vi "EQ_DATA_presort.vi"(8 "EQ Data and Report":u32[](array[numeric])=[2137719168, 671965161, 2137719168, 671965161, 2137719168, 671965161, 2137719168, 671965161, 2137719168, 671965161, 2137719168, 671965161, 2137719168, 671965161, 2137719168, 671965161, 2137719168, 671965161, 2137719168, 671965161, 2137719168, 671965161, 2137719168, 671965161, 2137719168, 671965161, 2137719168, 671965161, 2137719168, 671965161, 2137719168, 671965161, 2137719168, 671965161, 2137719168, 671965161, 2137719168, 671965161, 2137719168, 671965161, 2137719168, 671965161, 2137719168, 671965161, 2137719168, 671965161, 2137719168, 671965161, 2137719168, 671965161, 2137719168, 671965161, 2137719168, 671965161, 2137719168, 671965161, 2137719168, 671965161, 2137719168, 671965161, 2137719168, 671965161, 2137719168, 671965161, 2137719168, 671965161, 2137719168, 671965161, 2137719168, 671965161, 2137719168, 671965161, 2137719168, 671965161, 2137719168, 671965161, 2137719168, 671965161, 2137719168, 671965161, 2137719168, 671965161, 2137719168, 671965161, 2137719168, 671965161, 2137719168, 671965161, 2137719168, 671965161, 2137719168, 760049897, 2137719168, 491616745, 2137719168, 671965161, 2137719168, 671965161, 2137719168, 671965161, 2137719168, 671965161, 2137719168, 671965161, 2137719168, 671965161, 2137719168, 671965161, 2137719168, 671965161, 2137719168, 671965161, 2137719168, 671965161, 2137719168, 671965161, 2137719168, 671965161, 2137719168, 671965161, 2137719168, 671965161, 2137719168, 671965161, 2137719168, 671965161, 2137719168, 671965161, 2137719168, 671965161, 2137719168, 671965161, 2137719168, 671965161, 2137719168, 671965161, 2137719168, 671965161, 2137719168, 671965161, 2137719168, 671965161, 2137719168, 671965161, 2137719168, 671965161, 2137719168, 671965161, 2137719168, 671965161, 2137719168, 671965161, 2137719168, 671965161, 2137719168, 671965161, 2137719168, 671965161, 2137719168, 671965161, 2137719168, 671965161, 2137719168, 671965161, 2137719168, 671965161, 2137719168, 671965161, 2137719168, 671965161, 2137719168, 671965161, 2137719168, 671965161, 2137719168, 671965161, 2137719168, 671965161, 2137719168, 671965161, 2137719168, 671965161, 2137719168, 671965161, 2137719168, 671965161, 2137719168, 671965161, 2137719168, 671965161, 2137719168, 671965161, 2137719168, 671965161, 2137719168, 671965161, 2137719168, 671965161, 2137719168, 671965161, 2070610304, 671965161, 2070610304, 671965161, 2070610304, 671965161, 2070610304, 671965161, 2070610304, 671965161, 2070610304, 671965161, 2070610304, 671965161, 2070610304, 671965161, 2070610304, 671965161, 2070610304, 671965161, 2070610304, 671965161, 2070610304, 671965161, 2070610304, 671965161, 2070610304, 671965161, 2070610304, 671965161, 2070610304, 671965161, 2070610304, 671965161, 2070610304, 671965161, 2070610304, 671965161, 2070610304, 671965161, 2070610304, 671965161, 2070610304, 671965161, 2070610304, 671965161, 2070610304, 671965161, 2070610304, 671965161, 2070610304, 671965161, 2070610304, 671965161, 2070610304, 671965161, 2070610304, 671965161, 2070610304, 671965161, 2070610304, 671965161, 2070610304, 671965161, 2070610304, 671965161, 2070610304, 671965161, 2070610304, 671965161, 2070610304, 671965161, 2070610304, 671965161, 2070610304, 671965161, 2070610304, 671965161, 2070610304, 671965161, 2070610304, 671965161, 2070610304, 671965161, 2070610304, 671965161, 2070610304, 671965161, 2070610304, 671965161, 2070610304, 891148969, 2070610304, 1223555977, 2070610304, 671965161, 2070610304, 671965161, 2070610304, 671965161, 2070610304, 671965161, 2070610304, 671965161, 2070610304, 671965161, 2070610304, 671965161, 2070610304, 671965161, 2070610304, 671965161, 2070610304, 671965161, 2070610304, 671965161, 2070610304, 671965161, 2070610304, 671965161, 2070610304, 671965161, 2070610304, 671965161, 2070610304, 671965161, 2070610304, 671965161, 2070610304, 671965161, 2070610304, 671965161, 2070610304, 671965161, 2070610304, 671965161, 2070610304, 671965161, 2070610304, 671965161, 2070610304, 671965161, 2070610304, 671965161, 2070610304, 671965161, 2070610304, 671965161, 2070610304, 671965161, 2070610304, 671965161, 2070610304, 671965161, 2070610304, 671965161, 2070610304, 671965161, 2070610304, 671965161, 2070610304, 671965161, 2070610304, 671965161, 2070610304, 671965161, 2070610304, 671965161, 2070610304, 671965161, 2070610304, 671965161, 2070610304, 671965161, 2070610304, 671965161, 2070610304, 671965161, 2070610304, 671965161, 2070610304, 671965161, 2070610304, 671965161, 2070610304, 671965161, 2070610304, 671965161, 2070610304, 671965161, 2070610304, 671965161, 2070610304, 671965161, 2070610304, 671965161, 2070610304, 671965161, 2070610304, 671965161, 2104164736, 671965161, 2104164736, 671965161, 2104164736, 671965161, 2104164736, 671965161, 2104164736, 671965161, 2104164736, 671965161, 2104164736, 671965161, 2104164736, 671965161, 2104164736, 671965161, 2104164736, 671965161, 2104164736, 671965161, 2104164736, 671965161, 2104164736, 671965161, 2104164736, 671965161, 2104164736, 671965161, 2104164736, 671965161, 2104164736, 671965161, 2104164736, 671965161, 2104164736, 671965161, 2104164736, 671965161, 2104164736, 671965161, 2104164736, 671965161, 2104164736, 671965161, 2104164736, 671965161, 2104164736, 671965161, 2104164736, 671965161, 2104164736, 671965161, 2104164736, 671965161, 2104164736, 671965161, 2104164736, 671965161, 2104164736, 671965161, 2104164736, 671965161, 2104164736, 671965161, 2104164736, 671965161, 2104164736, 671965161, 2104164736, 671965161, 2104164736, 671965161, 2104164736, 671965161, 2104164736, 671965161, 2104164736, 671965161, 2104164736, 671965161, 2104164736, 671965161, 2104164736, 671965161, 2104164736, 671965161, 2104164736, 671965161, 2104164736, 691900489, 2104164736, 960314249, 2104164736, 671965161, 2104164736, 671965161, 2104164736, 671965161, 2104164736, 671965161, 2104164736, 671965161, 2104164736, 671965161, 2104164736, 671965161, 2104164736, 671965161, 2104164736, 671965161, 2104164736, 671965161, 2104164736, 671965161, 2104164736, 671965161, 2104164736, 671965161, 2104164736, 671965161, 2104164736, 671965161, 2104164736, 671965161, 2104164736, 671965161, 2104164736, 671965161, 2104164736, 671965161, 2104164736, 671965161, 2104164736, 671965161, 2104164736, 671965161, 2104164736, 671965161, 2104164736, 671965161, 2104164736, 671965161, 2104164736, 671965161, 2104164736, 671965161, 2104164736, 671965161, 2104164736, 671965161, 2104164736, 671965161, 2104164736, 671965161, 2104164736, 671965161, 2104164736, 671965161, 2104164736, 671965161, 2104164736, 671965161, 2104164736, 671965161, 2104164736, 671965161, 2104164736, 671965161, 2104164736, 671965161, 2104164736, 671965161, 2104164736, 671965161, 2104164736, 671965161, 2104164736, 671965161, 2104164736, 671965161, 2104164736, 671965161, 2104164736, 671965161, 2104164736, 671965161, 2104164736, 671965161, 2104164736, 671965161, 2104164736, 671965161, 2104164736, 671965161, 2104164736, 671965161, 2104164736, 671965161, 2028667264, 671965161, 2028667264, 671965161, 2028667264, 671965161, 2028667264, 671965161, 2028667264, 671965161, 2028667264, 671965161, 2028667264, 671965161, 2028667264, 671965161, 2028667264, 671965161, 2028667264, 671965161, 2028667264, 671965161, 2028667264, 671965161, 2028667264, 671965161, 2028667264, 671965161, 2028667264, 671965161, 2028667264, 671965161, 2028667264, 671965161, 2028667264, 671965161, 2028667264, 671965161, 2028667264, 671965161, 2028667264, 671965161, 2028667264, 671965161, 2028667264, 671965161, 2028667264, 671965161, 2028667264, 671965161, 2028667264, 671965161, 2028667264, 671965161, 2028667264, 671965161, 2028667264, 671965161, 2028667264, 671965161, 2028667264, 671965161, 2028667264, 671965161, 2028667264, 671965161, 2028667264, 671965161, 2028667264, 671965161, 2028667264, 671965161, 2028667264, 671965161, 2028667264, 671965161, 2028667264, 671965161, 2028667264, 671965161, 2028667264, 671965161, 2028667264, 671965161, 2028667264, 671965161, 2028667264, 671965161, 2028667264, 671965161, 2028667264, 555604297, 2028667264, 689765225, 2028667264, 671965161, 2028667264, 671965161, 2028667264, 671965161, 2028667264, 671965161, 2028667264, 671965161, 2028667264, 671965161, 2028667264, 671965161, 2028667264, 671965161, 2028667264, 671965161, 2028667264, 671965161, 2028667264, 671965161, 2028667264, 671965161, 2028667264, 671965161, 2028667264, 671965161, 2028667264, 671965161, 2028667264, 671965161, 2028667264, 671965161, 2028667264, 671965161, 2028667264, 671965161, 2028667264, 671965161, 2028667264, 671965161, 2028667264, 671965161, 2028667264, 671965161, 2028667264, 671965161, 2028667264, 671965161, 2028667264, 671965161, 2028667264, 671965161, 2028667264, 671965161, 2028667264, 671965161, 2028667264, 671965161, 2028667264, 671965161, 2028667264, 671965161, 2028667264, 671965161, 2028667264, 671965161, 2028667264, 671965161, 2028667264, 671965161, 2028667264, 671965161, 2028667264, 671965161, 2028667264, 671965161, 2028667264, 671965161, 2028667264, 671965161, 2028667264, 671965161, 2028667264, 671965161, 2028667264, 671965161, 2028667264, 671965161, 2028667264, 671965161, 2028667264, 671965161, 2028667264, 671965161, 2028667264, 671965161, 2028667264, 671965161, 2028667264, 671965161, 2028667264, 671965161, 2028667264, 671965161, 0, 0, 0, 0, 2137719295, 4294967295, 4294967295, 4294967264, 235670073, 68228136, 2070610431, 4294967295, 4294967295, 4294967264, 235670073, 68228136, 2104164863, 4294967295, 4294967295, 4294967264, 235670073, 68228136, 2028667391, 4294967295, 4294967295, 4294967264, 235670073, 68228136, 2137718784, 4293787621, 59180718, 2137718785, 262139, 58525283, 2137718786, 58525283, 58525283, 2137718787, 58525283, 58525283, 2137718788, 58525283, 58525283, 2137718789, 58525283, 58525283, 2137718790, 58525283, 58525283, 2137718791, 58525283, 58525283] format="%x", 9 "number of pixels":u32, 11 "Chip ID list":u32[](array[numeric]) format="%x") -> (2 "Data+Report ordLayers":u32[][](array[numeric]) format="%x")   [LabVIEW 2015, in "VIPM2.lvlib"]
doc: "Pre endreza les Layers per despres fer els Chip files."
uses:
  VIPM2.lvlib
panel:
  out "quants":i32[](array[numeric])
  # "Si Layer = FFFF, pre endreza les Layers per despres fer els Chip files"
  # "row: DATA+REPORT 1 Layer"
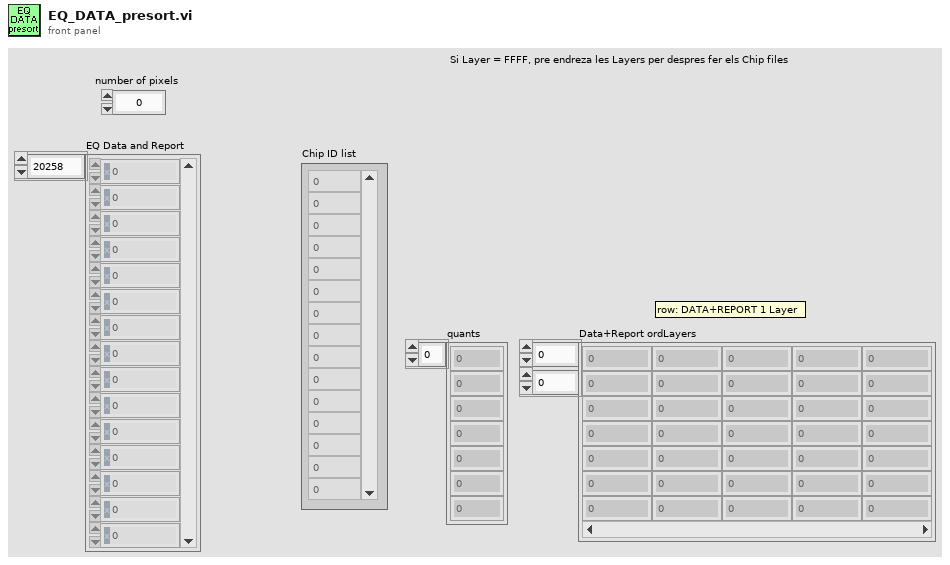
[diagram p1: front panel]
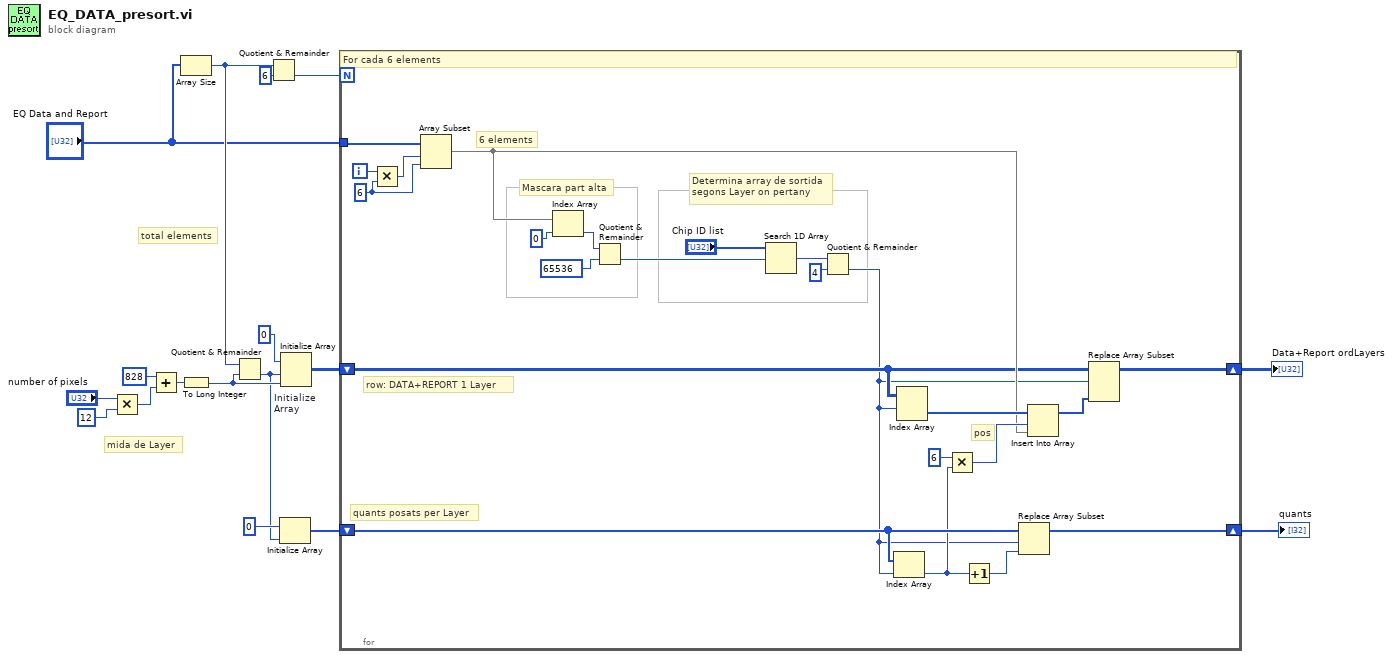
[diagram p0: block diagram]
diagram:
  # "mida de Layer"
  # "total elements"
  n1 = Multiply(x="number of pixels", y=u32 12) -> (x*y=w9:u32)
  n2 = Add(x=u32 828 ("dimension size"), y=w9) -> (x+y=w7:u32)
  n3 = Array Size(array="EQ Data and Report") -> (size(s)=w8:i32)
  n4 = To Long Integer(number=w7) -> (32bit integer=w6:i32)
  n5 = Quotient & Remainder(x=w8, y=w6) -> (floor(x/y)=w3:i32)  [unwired: 1 out]
  n6 = Quotient & Remainder(x=w8, y=6) -> (floor(x/y)=w16:i32)  [unwired: 1 out]
  n7 = Initialize Array(0 ("y"), w3) -> (w5:i32[])
  n8 = Initialize Array "Initialize\nArray"(u32 0 ("dimension size"), w3, w6) -> (w14:u32[][])
  n9 = for {
    N: w16 -> [_]
    tunnel: "EQ Data and Report" -> [w39]
    shift-right: [w23] -> w2
    shift-left: w14 -> [w24]
    shift-right: [w19] -> w15
    shift-left: w5 -> [w22]
    i -> [w40]
    w37 = 6 ("y")
    # "row: DATA+REPORT 1 Layer"
    # "pos"
    # "Determina array de sortida\nsegons Layer on pertany"
    # "quants posats per Layer"
    # "Mascara part alta"
    # "6 elements"
    # "For cada 6 elements"
    n10 = Multiply(x=w40, y=w37) -> (x*y=w38:i32)
    n11 = Array Subset "Array Subset"(array=w39, index=w38, length=w37) -> (w26:u32[])
    n12 = Index Array(array=w26, index=0) -> (element=w34:u32)
    n13 = Quotient & Remainder(x=w34, y=u32 65536) -> (floor(x/y)=w33:u32)  [unwired: 1 out]
    n14 = Search 1D Array(1D array="Chip ID list", element=w33) -> (index of element=w31:i32)  [unwired: 1 in]
    n15 = Quotient & Remainder(x=w31, y=4) -> (floor(x/y)=w18:i32)  [unwired: 1 out]
    n16 = Index Array "Index Array"(array=w22, index=w18) -> (element=w20:i32)
    n17 = Index Array "Index Array"(array=w24, index (row)=w18) -> (element=w28:u32[])  [unwired: 1 in]
    n18 = Multiply(x=6, y=w20) -> (x*y=w27:i32)
    n19 = Increment(x=w20) -> (x+1=w21:i32)
    n20 = Replace Array Subset "Replace Array Subset"(array=w22, new element=w21, index=w18) -> (w19:i32[])
    n21 = Insert Into Array "Insert Into Array"(array=w28, index=w27, new element=w26) -> (w25:u32[])
    n22 = Replace Array Subset "Replace Array Subset"(array=w24, new element=w25, index (row)=w18) -> (w23:u32[][])  [unwired: 1 in]
  }
  "quants" <- w15
  "Data+Report ordLayers" <- w2
